vi "FTW-CodeGen-JSON-GetTerms4.vi"(0 "State In":T2, 5 "XRef":refnum<vi>) -> (4 "Terms":T1(array[cluster]))   [LabVIEW 2012, in "FTW-JSON-Deserialize.xnode"]
uses:
  src/JSON/FTW-JSON-Deserialize.xnode
  FTW-CodeGen-JSON-State.ctl
panel:
  # "Inputs"
  # "Outputs"
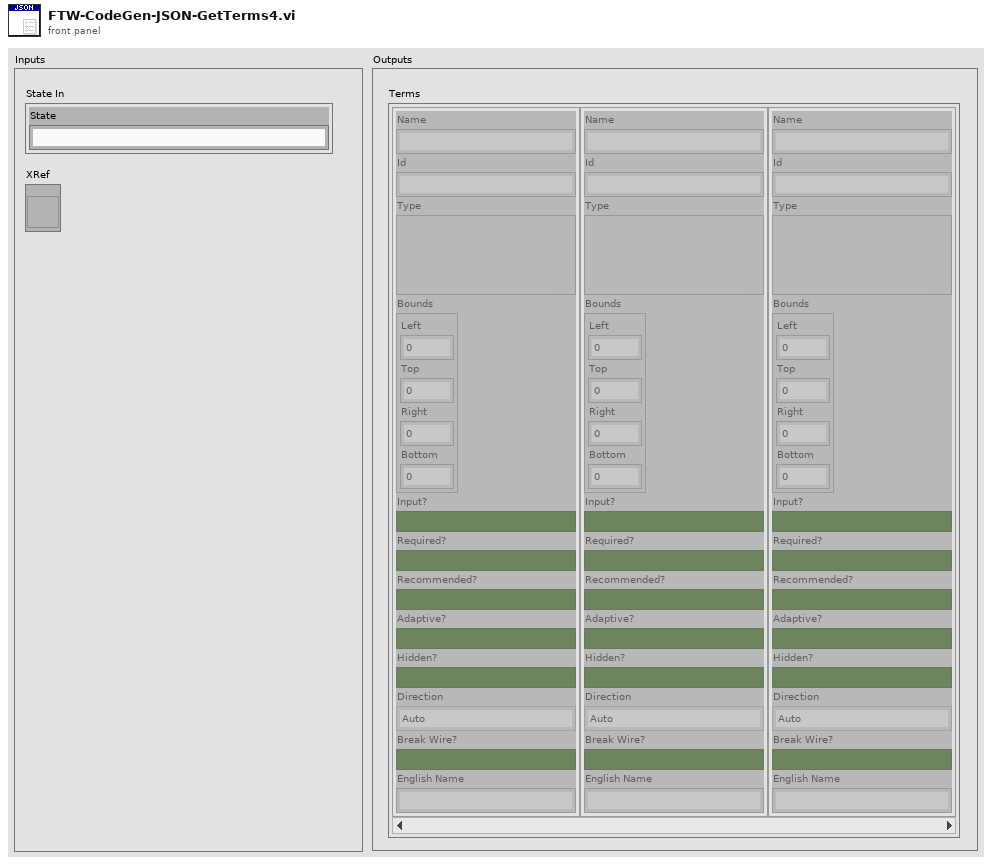
[diagram p1: front panel]
types:
  T1 = cluster{"Name":string, "Id":string, "Type":variant, "Bounds":cluster{"Left":i32, "Top":i32, "Right":i32, "Bottom":i32}, "Input?":bool, "Required?":bool, "Recommended?":bool, "Adaptive?":bool, "Hidden?":bool, "Direction":enum32{"Auto", "Up", "Down", "Left", "Right", "Center"}, "Break Wire?":bool, "English Name":string}[]
  T2 = typedef "FTW-JSON-Deserialize.xnode/FTW-CodeGen-JSON-State.ctl" = cluster{"State":string}
  T3 = cluster{"Left":i32, "Top":i32, "Right":i32, "Bottom":i32}[]
  T4 = cluster{"Name":string, "Id":string, "Type":variant, "Bounds":cluster{"Left":i32, "Top":i32, "Right":i32, "Bottom":i32}, "Input?":bool, "Required?":bool, "Recommended?":bool, "Adaptive?":bool, "Hidden?":bool, "Direction":enum32{"Auto", "Up", "Down", "Left", "Right", "Center"}, "Break Wire?":bool, "English Name":string}
  T5 = typedef "LVRectTypeDef.ctl" = cluster{"Left":i16, "Top":i16, "Right":i16, "Bottom":i16}
  T6 = enum16{"Invalid Wire Rule", "Required", "Recommended", "Optional", "Dynamic Dispatch"}[]
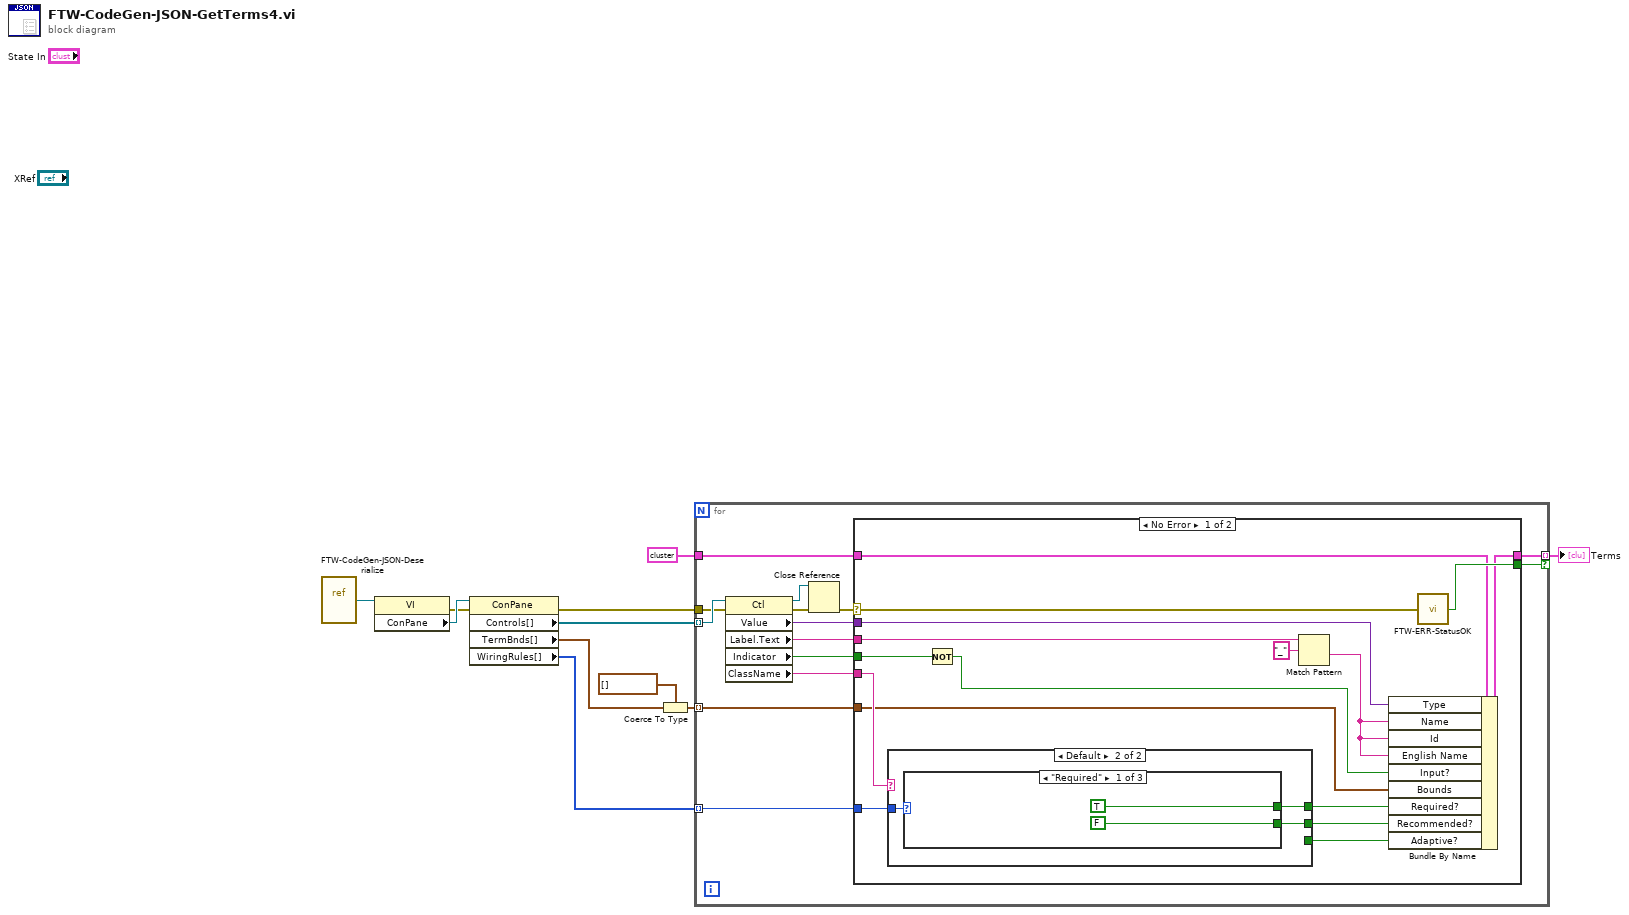
[diagram p0: block diagram]
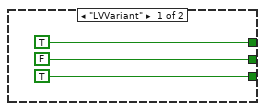
[diagram p2: hidden frame]
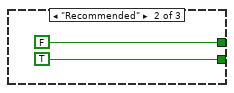
[diagram p3: hidden frame]
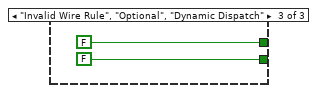
[diagram p4: hidden frame]
diagram:
  n1 = vi-ref "FTW-CodeGen-JSON-Deserialize.vi"() -> (w11:refnum<vi>)
  n2 = property class="VI"(reference=w11) -> (error out=w7:errorcluster, "ConPane"=w10:refnum<vi>)  [unwired: 1 in, 1 out]
  n3 = property class="ConPane"(reference=w10, error in=w7) -> (error out=w6:errorcluster, "Controls[]"=w9:refnum<vi>[], "TermBnds[]"=w3:T5[], "WiringRules[]"=w4:T6)  [unwired: 1 out]
  n4 = Coerce To Type(0:w3, 1:T3 []) -> (2:w1:T3)
  n5 = for {
    tunnel: w1 -> [w23] mode=indexing
    tunnel: w9 -> [w21] mode=indexing
    tunnel: w4 -> [w22] mode=indexing
    tunnel: T4 {"Name"="", "Id"="", "Type"=variant, "Bounds"={"Left"=0, "Top"=0, "Right"=0, "Bottom"=0}, "Input?"=FALSE, "Required?"=FALSE, "Recommended?"=FALSE, "Adaptive?"=FALSE, "Hidden?"=FALSE, "Direction"=enum."Auto", "Break Wire?"=FALSE, "English Name"=""} ("Term 4") -> [w25]
    tunnel: [w24] -> w8 mode=indexing if=w15
    tunnel: w6 -> [w16]
    n6 = property class="Ctl"(reference=w21, error in=w16) -> (reference out=w14:refnum<vi>, error out=w13:errorcluster, "Value"=w20:variant, "Label.Text"=w19:string, "Indicator"=w17:bool, "ClassName"=w18:string)
    n7 = Close Reference(reference=w14, error in (no error)=w13) -> (error out=w12:errorcluster)
    n8 = case shown="No Error" w12 {
      selector: w12 -> [w28 _]
      tunnel: w25 -> [w40 w54]
      tunnel: [w39 w54] -> w24
      tunnel: w23 -> [w27 _]
      tunnel: w22 -> [w38 _]
      tunnel: w20 -> [w35 _]
      tunnel: w18 -> [w34 _]
      tunnel: w19 -> [w31 _]
      tunnel: w17 -> [w32 _]
      tunnel: [w41 _] -> w15
      frame No Error {
        n9 = case shown="Default" w34 {
          tunnel: w38 -> [_ w47]
          tunnel: [TRUE w46] -> w37
          tunnel: [FALSE w45] -> w36
          tunnel: [TRUE _] -> w33
          frame "LVVariant" {
          }
          frame Default {
            n10 = case shown="\"Required\"" w47 {
              tunnel: [TRUE FALSE FALSE] -> w46
              tunnel: [FALSE TRUE FALSE] -> w45
              frame "Required" {
              }
              frame "Recommended" {
              }
              frame "Invalid Wire Rule", "Optional", "Dynamic Dispatch" {
              }
            }
          }
        }
        n11 = Not(x=w32) -> (.not. x?=w26:bool)
        n12 = Match Pattern(string=w31, regular expression="_") -> (after substring=w29:string)  [unwired: 1 in, 3 out]
        n13 = Bundle By Name(cluster=w40, "Type"=w35, "Name"=w29, "Id"=w29, "English Name"=w29, "Input?"=w26, "Bounds"=w27, "Required?"=w37, "Recommended?"=w36, "Adaptive?"=w33) -> (w39:T4)
        n14 = call "FTW-ERR-StatusOK.vi"("error to check"=w28) -> ("Status OK?"=w41:bool)
      }
      frame Error {
      }
    }
  }
  "Terms" <- w8
